vi "Stop.vi"(8 "error in (no error)":errorcluster) -> (0 "error out":errorcluster)   [LabVIEW 2020, in "Manipulator CLI Driver.lvlib"]
uses:
  Manipulator CLI Driver.lvlib
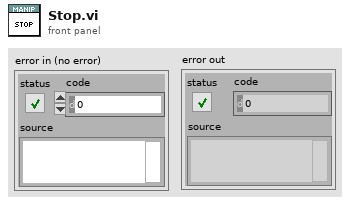
[diagram p1: front panel]
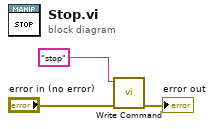
[diagram p0: block diagram]
diagram:
  n1 = call "Write Command.vi"("error in (no error)"="error in (no error)", "command"="stop") -> ("error out"=→"error out":errorcluster)  [unwired: 7 in, 2 out]
